vi "shutdown_time_input.vi"() -> (4 "delta value output":dbl, 10 "Done output":bool, 15 "Finish output":bool)   [LabVIEW 2018]
panel:
  in  "Finish":bool
  in  "Delta":string caption="\"y\" value"
  # "Laser Shutdown"
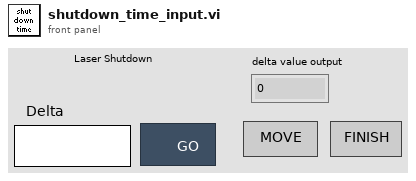
[diagram p1: front panel]
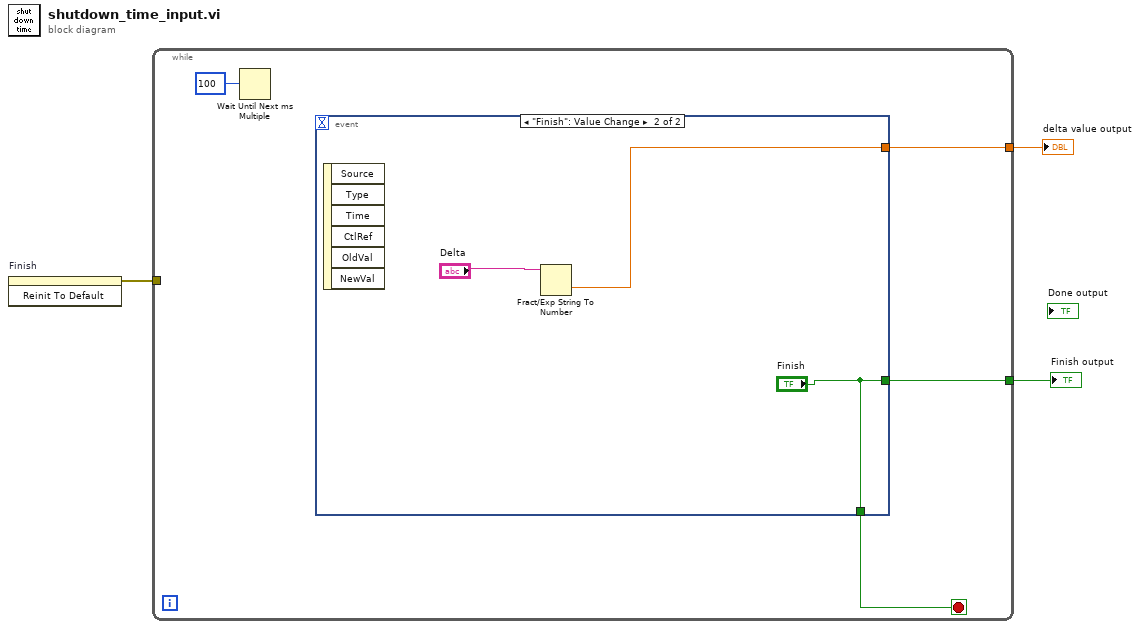
[diagram p0: block diagram]
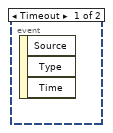
[diagram p2: hidden frame]
diagram:
  n1 = invoke on="Finish" class="Bool" method="Reinit To Default"() -> (error out=w3:errorcluster)  [unwired: 3 in, 2 out]
  n2 = while {
    tunnel: [w6] -> w2
    tunnel: w3 -> [_]
    tunnel: [w5] -> w1
    stop <- w4 stop-if-true
    n3 = Wait Until Next ms Multiple(millisecond multiple=100) -> ()  [unwired: 1 out]
    n4 = event shown="[1] \"Finish\": Value Change" {
      selector: _ -> [_ _]
      dyn-events: _ -> [_ _]
      timeout: _ -> [_ _]
      tunnel: [_ w8] -> w6
      tunnel: [_ "Finish"] -> w5
      tunnel: [_ "Finish"] -> w4
      event Timeout {
        n5 = event-data() -> ()  [unwired: 1 in, 3 out]
      }
      event "Finish": Value Change {
        n6 = event-data() -> ()  [unwired: 1 in, 6 out]
        n7 = Fract/Exp String To Number(string="Delta") -> (number=w8:dbl)  [unwired: 3 in, 1 out]
      }
    }
  }
  "delta value output" <- w2
  "Finish output" <- w1
